vi "unix time 1ms.vi"() -> (0 "time stamp":timestamp, 1 "unix time (ms)":u64)   [LabVIEW 2019, in "Timers.lvlib"]
uses:
  Timers.lvlib
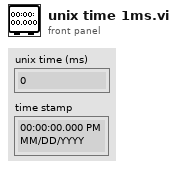
[diagram p1: front panel]
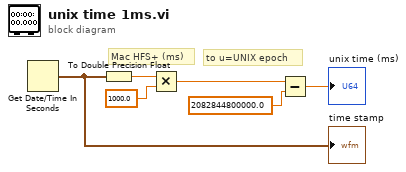
[diagram p0: block diagram]
diagram:
  # "to u=UNIX epoch"
  # "Mac HFS+ (ms)"
  n1 = Get Date/Time In Seconds() -> (seconds since 1Jan1904=w2:timestamp)
  "time stamp" <- w2
  n2 = To Double Precision Float(number=w2) -> (double precision float=w5:dbl)
  n3 = Multiply(x=w5, y=1000.0) -> (x*y=w3:dbl)
  n4 = Subtract(x=w3, y=2082844800000.0) -> (x-y=→"unix time (ms)":dbl)
